vi "DataStream_PC_Read.vi"(4 "Point Size":i32, 6 "Milliseconds To Wait":u32, 7 "Map":map{string, T1}(c390), 8 "Error":errorcluster, 11 "Stream Ref":T2) -> (0 "Error Out":errorcluster, 1 "New Update Out":bool, 2 "Connected Out":bool, 3 "Stream Ref Out":T2, 5 "Map Out":map{string, T1}(c390))   [LabVIEW 2023]
uses:
  TypeDefs/Cluster_DataStream_PC Reader Refs.ctl
  TypeDefs/Cluster_DataStream PC Map Data Set.ctl
  <resource>/objmgr/ni.dex.rc
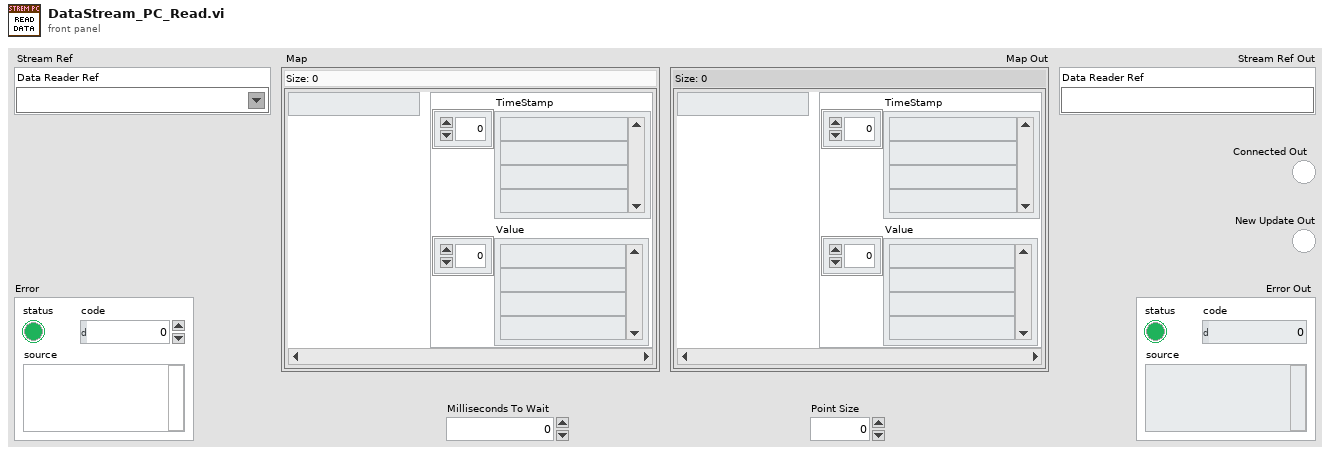
[diagram p1: front panel]
types:
  T1 = typedef "Cluster_DataStream PC Map Data Set.ctl" = cluster{"TimeStamp":dbl[], "Value":dbl[]}
  T2 = typedef "Cluster_DataStream_PC Reader Refs.ctl" = cluster{"Data Reader Ref":refnum<k21>}
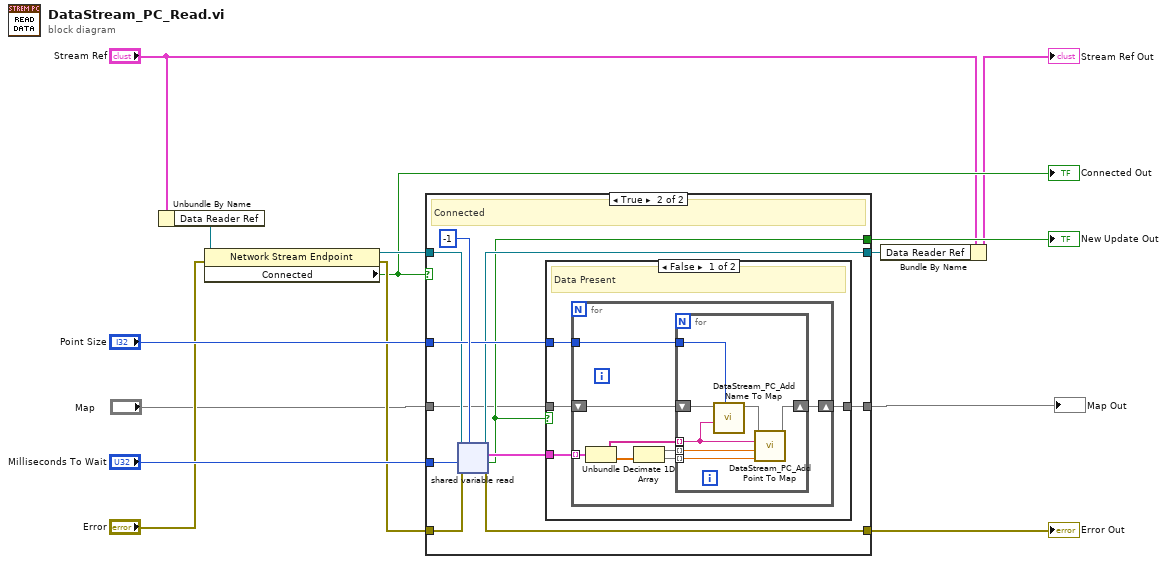
[diagram p0: block diagram]
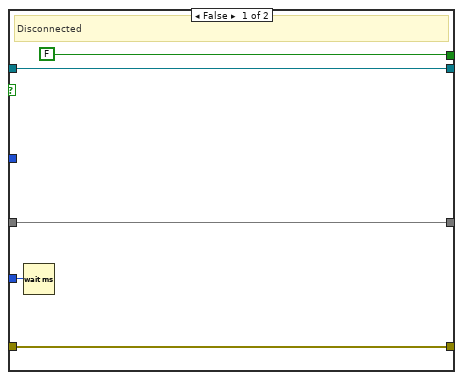
[diagram p2: hidden frame]
diagram:
  n1 = Unbundle By Name("Stream Ref") -> ("Data Reader Ref"=w7:refnum<k21>)
  n2 = property class="Network Stream Endpoint"(reference=w7, error in="Error") -> (reference out=w10:refnum<k21>, error out=w11:errorcluster, "Connected"=w9:bool)
  "Connected Out" <- w9
  n3 = case shown="True" w9 {
    tunnel: [w15 w30] -> w8
    tunnel: [FALSE w21] -> w14
    tunnel: "Milliseconds To Wait" -> [w18 w28]
    tunnel: "Point Size" -> [_ w27]
    tunnel: [w16 w26] -> w1
    tunnel: [w17 w25] -> w6
    tunnel: w11 -> [w16 w24]
    tunnel: w10 -> [w17 w23]
    tunnel: "Map" -> [w15 w20]
    frame False {
      # "Disconnected"
      n4 = Wait (ms)(milliseconds to wait=w18) -> ()  [unwired: 1 out]
    }
    frame True {
      # "Connected"
      n5 = shared-variable-read(w23, w24, w28, -1 ("# elements")) -> (w25:refnum<k21>, w26:errorcluster, w21:bool, w22:cluster{string[], dbl[]}[])
      n6 = case shown="False" w21 {
        tunnel: [w34 w50] -> w30
        tunnel: w27 -> [w33 _]
        tunnel: w20 -> [w32 w50]
        tunnel: w22 -> [w31 _]
        frame False {
          # "Data Present"
          n7 = for {
            tunnel: w33 -> [w41]
            tunnel: w31 -> [w39] mode=indexing
            shift-right: [w42] -> w34
            shift-left: w32 -> [w40]
            n8 = Unbundle(w39) -> (w38:string[], w37:dbl[])
            n9 = Decimate 1D Array(w37) -> (w36:dbl[], w35:dbl[])
            n10 = for {
              tunnel: w41 -> [w44]
              shift-right: [w49] -> w42
              shift-left: w40 -> [w45]
              tunnel: w38 -> [w43] mode=indexing
              tunnel: w36 -> [w48] mode=indexing
              tunnel: w35 -> [w47] mode=indexing
              n11 = call "DataStream_PC_Add Name To Map.vi"("Point Size"=w44, "Name"=w43, "Map"=w45) -> ("Map Out"=w46:map{string, T1})  [unwired: 8 in]
              n12 = call "DataStream_PC_Add Point To Map.vi"("Value"=w47, "Time Stamp"=w48, "Name"=w43, "Map"=w46) -> ("Map Out"=w49:map{string, T1})  [unwired: 7 in]
            }
          }
        }
        frame True {
          # "Not Data"
        }
      }
    }
  }
  "New Update Out" <- w14
  "Error Out" <- w1
  "Map Out" <- w8
  n13 = Bundle By Name(cluster="Stream Ref", "Data Reader Ref"=w6) -> (→"Stream Ref Out":T2)
